vi "Dust_Source_Control_small.vi"(7 "error in":errorcluster) -> (0 "error out":errorcluster)   [LabVIEW 2013]
doc: "This VI specifies the properties of the pulse used for running the dust source. When program is stopped, the voltage is incrementally reduced to zero to avoid quick drops."
uses:
  <vilib>/Utility/miscctls.llb/LVPointTypeDef.ctl
  Global Variables/Action Items.ctl
  <vilib>/Utility/error.llb/DialogType.ctl
  <vilib>/DAQmx/read.llb/DAQmx Read (Analog 1D Wfm NChan NSamp).vi
  <vilib>/Analysis/baseanly.llb/Mean (DBL).vi
  <vilib>/DAQmx/write.llb/DAQmx Write (Analog 1D Wfm NChan NSamp).vi
  <vilib>/DAQmx/read.llb/DAQmx Read (Counter U32 1Chan 1Samp).vi
  <vilib>/DAQmx/create/channels.llb/DAQmx Create Channel (AI-Voltage-Basic).vi
  <vilib>/DAQmx/configure/timing.llb/DAQmx Timing (Sample Clock).vi
  <vilib>/DAQmx/create/channels.llb/DAQmx Create Channel (AO-Voltage-Basic).vi
  <vilib>/DAQmx/create/channels.llb/DAQmx Create Channel (CI-Count Edges).vi
  <userlib>/_OpenG.lib/comparison/comparison.llb/DBL Changed__ogtk.vi
  <vilib>/measure/mascope.llb/Amplitude and Levels 1 chan.vi
  <vilib>/DAQmx/miscellaneous.llb/DAQmx Fill In Error Info.vi
  Global Variables/throttle.vi
  <userlib>/_OpenG.lib/comparison/comparison.llb/Boolean Changed__ogtk.vi
  Global Variables/throttle from query.vi
  Sub-Polymorphic/post_run_times.vi
  Sub-Polymorphic/update_counter_entry_small.vi
  Sub-Polymorphic/post_dust_event_big.vi
  Sub-Polymorphic/post_dust_source_small.vi
  <vilib>/addons/database/_DB Variant To Data/Database Variant To Data.xnode
  <resource>/objmgr/daqmx.rc
  <vilib>/measure/NI_MAPro.lvlib
  <vilib>/Analysis/NI_AALBase.lvlib
panel:
  out "Freq. Before Throttle":dbl
  out "On/Off":bool
  out "Finished":bool=TRUE
  out "Output waveform":waveform(dbl)={"t0"=timestamp(0 s since 1904-01-01), "dt"=4e-06, "Y"=array[50000 elements]}
  out "Input waveform":waveform(dbl)={"t0"=timestamp(3437998856.0330505 s since 1904-01-01), "dt"=0.00019999999999999998, "Y"=array[1000 elements], "attributes"=variant("NI_ChannelName"=variant(string "Dev5/ai20"), "NI_UnitDescription"=variant(string "Volts"))}
  out "output cluster":T1={"Integer Timestamp"=0, "Needle Voltage"=0.0, "Frequency"=1.0, "Width (ms) : 0.1 "=0.1, "Desired Amplitude (V)"=0.0, "Settings ID"="", "ID#"=0} {"Needle Voltage" min=0.0 max=10.0 step=0.01 format="%.2g"; "Desired Amplitude (V)" min=0.0 max=10.0 step=0.01 format="%5.2f"; "Width (ms) : 0.1" min=0.05 max=5.0 step=0.01 format="%6.2f"; "Frequency" min=1.0 max=100.0 step=0.01 format="%.1f"}
  in  "Tab Control":enum32{"Controls", "Status", "Counter"}(tab)
  in  "Big Accelerator\nSetting?":bool
  out "Actual output width (ms)":dbl caption="Actual Output Width (ms)" format="%.2f"
  out "Actual output Frequency":dbl caption="Actual Output  Frequency (hz)" format="%.2f"
  in  "Width (ms) : 0.1":dbl=0.1 min=0.0 max=5.0 step=0.01 format="%6.2f"
  out "Actual Amplitude (V) 2":dbl=0.0012999050305587314 caption="Actual Amplitude (V)" format="%.2f"
  in  "Desired Amplitude (V)":dbl min=0.0 max=10.0 step=0.01 format="%5.2f"
  out "Actual output Amplitude (V)":dbl caption="Actual Output Amplitude (V)" format="%.2f"
  in  "Frequency":dbl=1.0 caption="Frequency (Hz) : 1" min=0.0 max=30.0 step=0.01 format="%.1f"
  in  "Abort Change":bool
  out "Actual Needle (kV)":dbl=-1.1093266413053247 caption="Actual Einzel (V)" format="%.2f"
  out "Actual Needle Output (V)":dbl caption="Actual Einzel (V)" format="%.2f"
  in  "Needle Voltage":dbl min=0.0 max=10.0 step=0.01 format="%.2g"
  in  "Save Settings?":bool
  out "CONTROLS":waveform(dbl)[](graph)=[{"t0"=timestamp(0 s since 1904-01-01), "dt"=4e-06, "Y"=array[50000 elements]}, {"t0"=timestamp(3437998856.0330505 s since 1904-01-01), "dt"=0.00019999999999999998, "Y"=array[1000 elements], "attributes"=variant("NI_ChannelName"=variant(string "Dev5/ai20"), "NI_UnitDescription"=variant(string "Volts"))}]
  in  "Settings ID":string
  in  "Retrieve Settings":bool
  out "Ratio of particles at\nsecond detector to first":dbl
  out "First detector since\nlast source change:":i64
  out "Average Rate of first":dbl
  out "Average Rate of second":dbl
  in  "# of Cycles ot Average":i32=10
  out "Number of Hours":dbl
  out "Chamber Pressure":dbl format="%#_3g"
  in  "Physical Channels":tag="Dev4/ao0:1" caption="Physical Output Channels"
  in  "Physical Input Channels":tag="Dev6/ai0:2"
  out "Execution Number:":i32=341
  out "Testing":bool
  in  "Counters On/Off":bool=TRUE
  in  "Reset Counters":bool
  in  "Det1":tag="Dev5/ctr0"
  in  "Det2":tag="Dev5/ctr1"
  out "Det2":u32
  out "Det1":u32
  out "error?":bool
  out "Actual Sample Clock Rate":dbl=250000.0 format="%.2f"
  in  "stop":bool
  # "CCLDAS Dust Control Small Accelerator"
  # "Hold Down to\nStop Changes"
  # "Tube Drive (Ao0, Ai4)"
  # "Needle Control (Ao4, Ai0)"
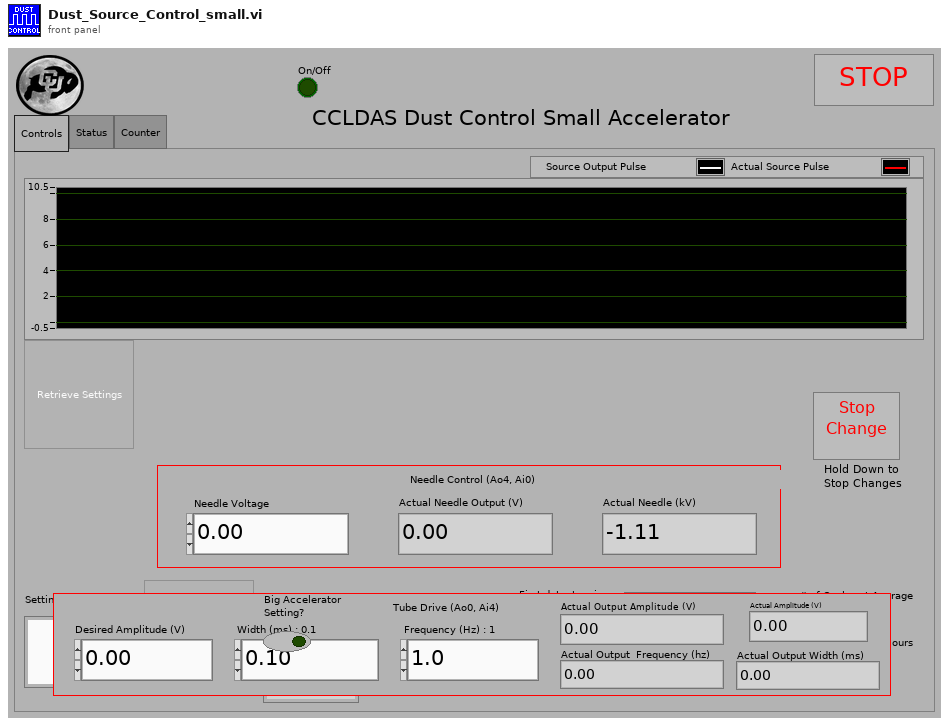
[diagram p1: front panel]
types:
  T1 = cluster{"Integer Timestamp":u64, "Needle Voltage":dbl, "Frequency":dbl, "Width (ms) : 0.1 ":dbl, "Desired Amplitude (V)":dbl, "Settings ID":string, "ID#":i32}
  T2 = typedef "Action Items.ctl" = enum16{"Initialize", "Get", "Set"}
  T3 = typedef "LVPointTypeDef.ctl" = cluster{"Horizontal":i16, "Vertical":i16}
  T4 = enum8{"Enabled", "Disabled", "Disabled and Grayed Out"}
  T5 = typedef "DialogType.ctl" = u16
  T6 = typedef "dust_source_control.ctl" = cluster{"Integer Timestamp":u64, "Einzel Voltage":dbl, "Needle Voltage":dbl, "Frequency":dbl, "Width (ms) : 0.1 ":dbl, "Desired Amplitude (V)":dbl, "X Voltage":dbl, "Y Voltage":dbl, "Settings ID":string, "ID#":i32}
  T7 = cluster{"Integer Time":i64, "Integer Time":i64, "Experiment ID":i64}
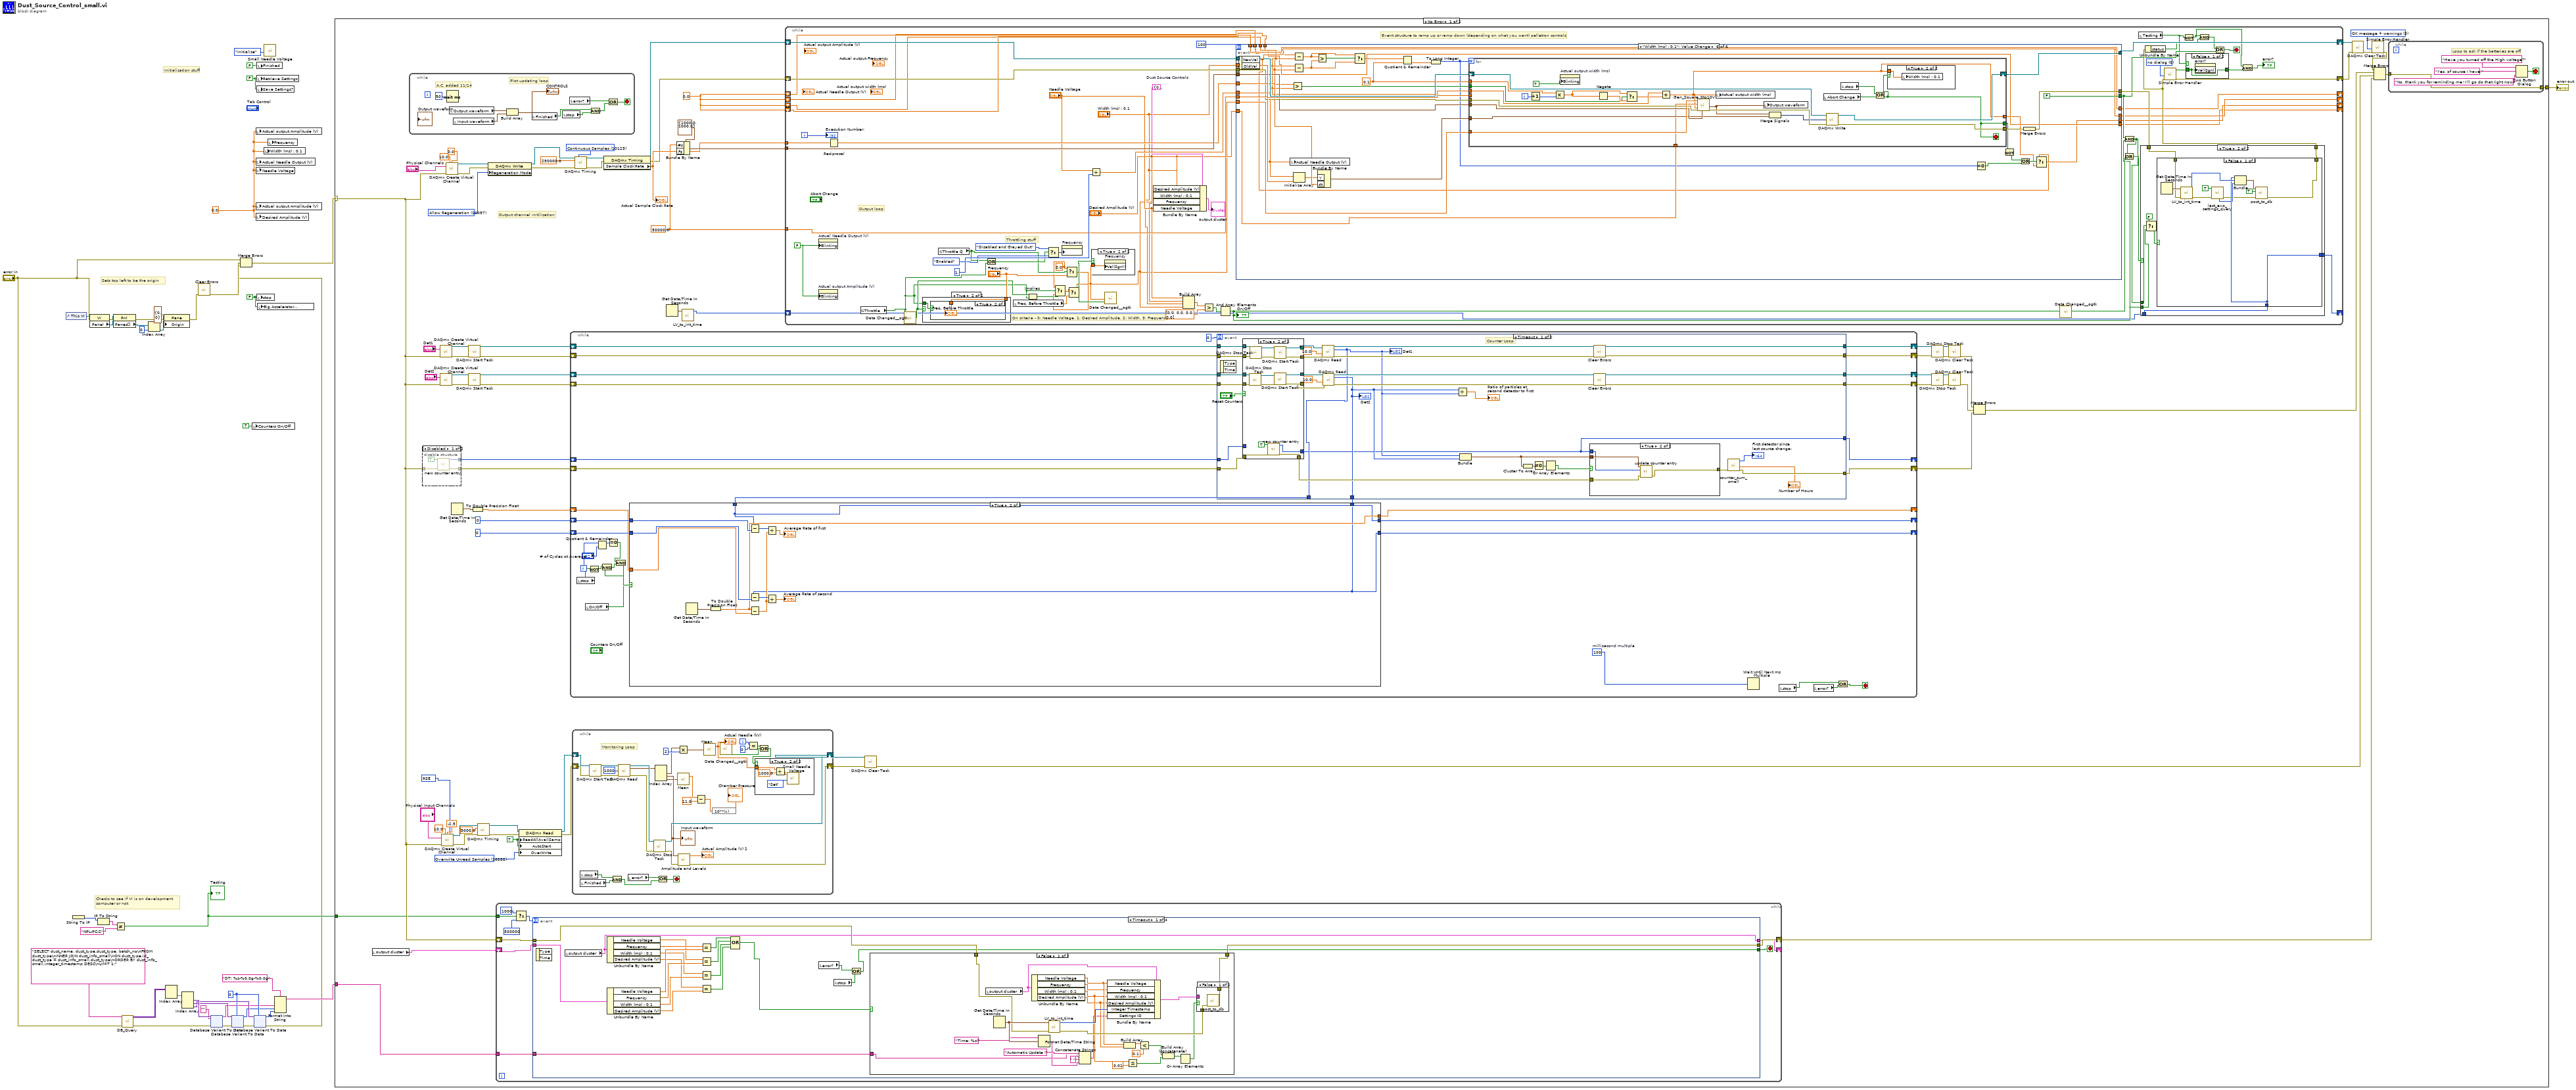
[diagram p0: block diagram]
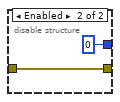
[diagram p2: hidden frame]
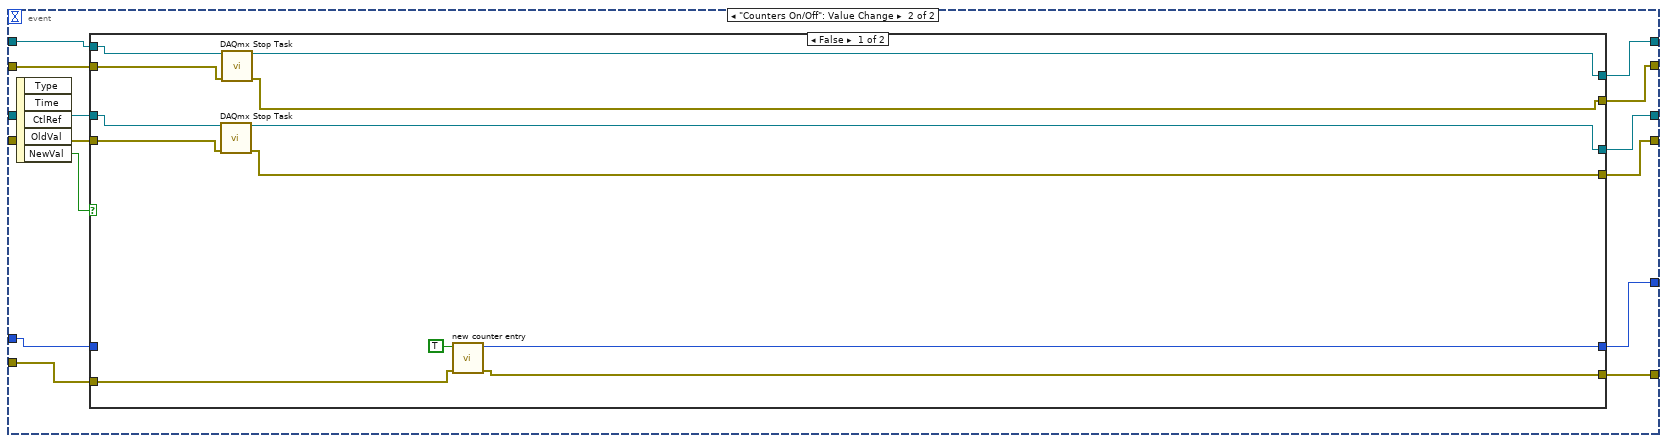
[diagram p5: hidden frame]
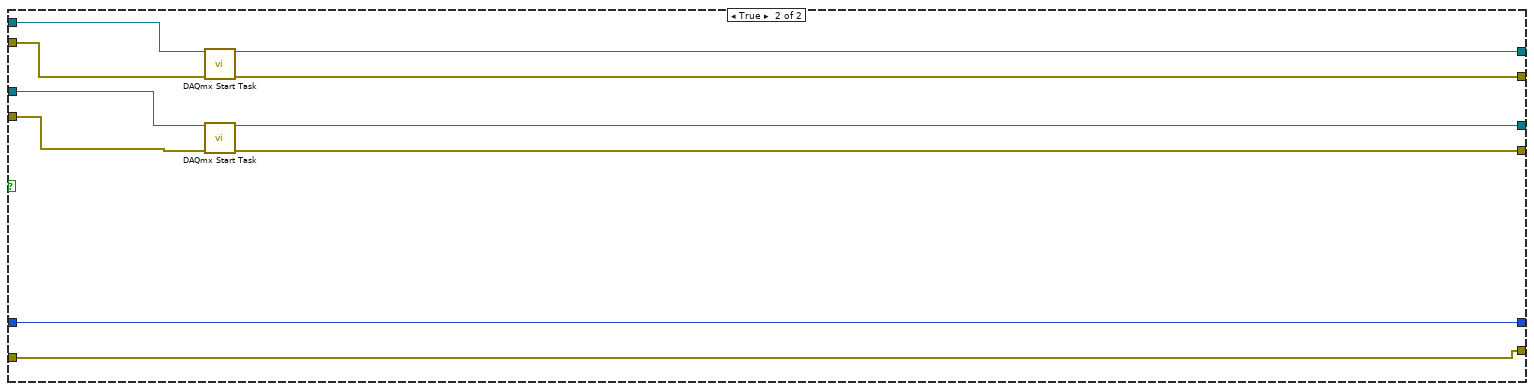
[diagram p6: hidden frame]
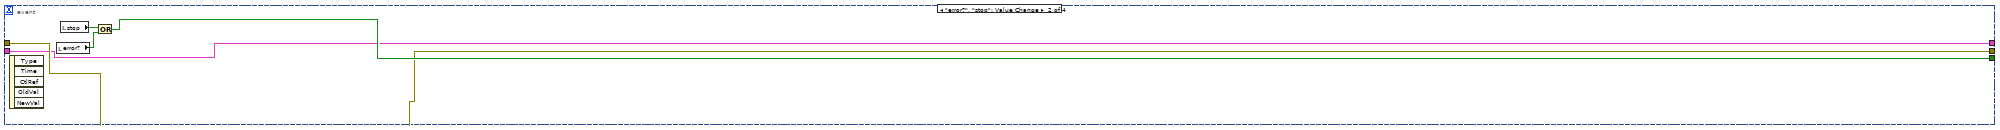
[diagram p11: hidden frame]
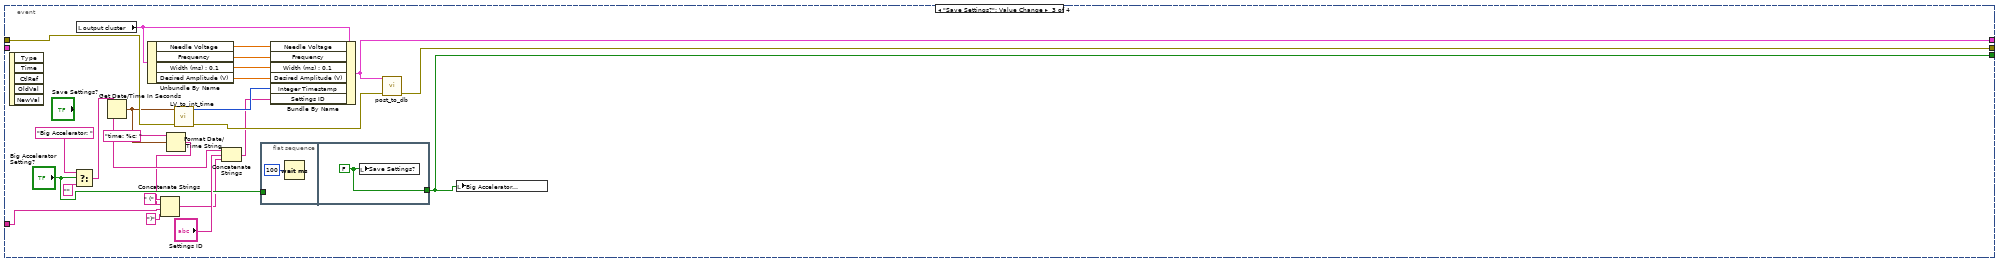
[diagram p12: hidden frame]
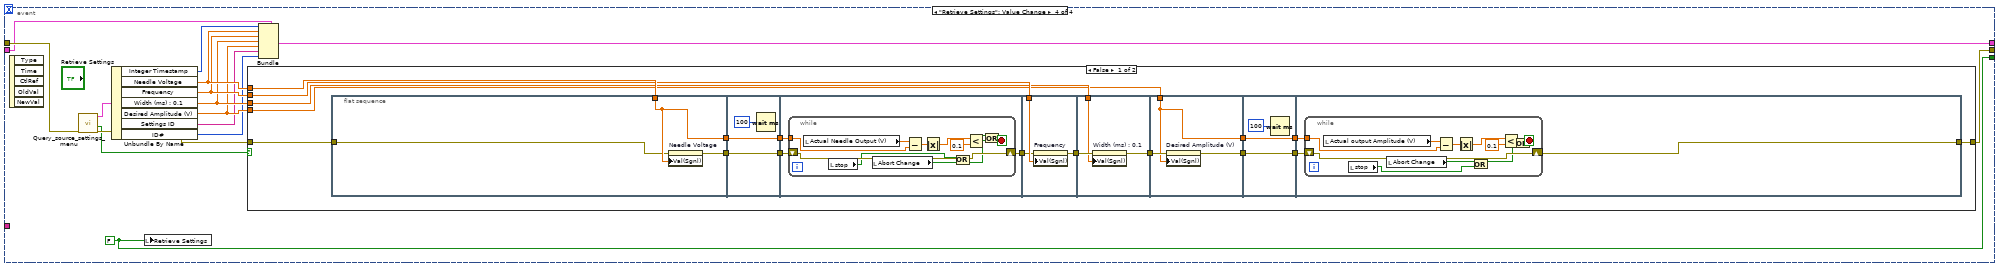
[diagram p13: hidden frame]
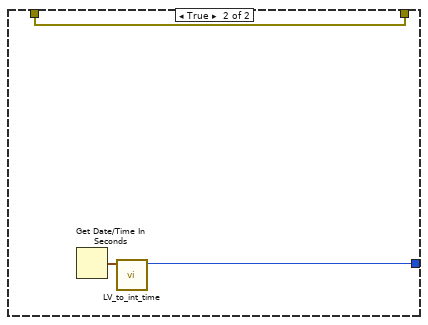
[diagram p19: hidden frame]
diagram:
  w16 = 0
  w38 = FALSE ("Retrieve Settings")
  w36 = 0.0 ("Actual Output (V)")
  w35 = FALSE ("Shutdown")
  # "Checks to see if VI is on development\ncomputer or not"
  # "Sets top left to be the origin"
  # "Initialization stuff"
  n1 = control-ref of="This VI"() -> (w34:refnum<vi>)
  n2 = String To IP() -> (0:w26:u32)  [unwired: 1 in]
  n3 = property class="VI"(reference=w34, error in="error in") -> (error out=w33:errorcluster, "Panel"=w32:refnum<vi>)  [unwired: 1 out]
  n4 = IP To String(2:w26) -> (0:w25:string)  [unwired: 1 in]
  n5 = property class="Pnl"(reference=w32, error in=w33) -> (error out=w31:errorcluster, "Panes[]"=w30:refnum<vi>[])  [unwired: 1 out]
  n6 = Not Equal?(x=w25, y="NPL-PC-2") -> (x != y?=w10:bool)
  "Testing" <- w10
  n7 = call "DB_Query.vi"("error in (no error)"="error in", "Parameterized Query"="SELECT dust_name, dust_type.dust_type, batch_no\nFROM dust_type\nINNER JOIN dust_info_small\nON dust_type.id_dust_type = dust_info_small.dust_type\nORDER BY dust_info_small.integer_timestamp DESC\nLIMIT 1;" ("SQL query")) -> ("error out"=w4:errorcluster, "Results"=w3:variant[][])  [unwired: 7 in, 1 out]
  n8 = Index Array(array=w30, index=0) -> (element=w28:refnum<vi>)
  n9 = property class="Pane"(reference=w28, error in=w31, "Origin"=T3 {"Horizontal"=0, "Vertical"=0}) -> (error out=w7:errorcluster)  [unwired: 1 out]
  n10 = Index Array(array=w3) -> (element=w23:variant[])  [unwired: 2 in]
  n11 = Index Array(array=w23) -> (element #1=w22:variant, element #2=w19:variant, element #3=w18:variant)  [unwired: 3 in]
  n12 = call <vilib>:"Clear Errors.vi"("error in (no error)"=w7) -> ("error out"=w8:errorcluster)  [unwired: 6 in]
  n13 = xnode "Database Variant To Data"("database variant"=w22, "error in (no error)"=w4, "type"="") -> ("data"=w14:string, "error out"=w21:errorcluster)
  n14 = xnode "Database Variant To Data"("database variant"=w19, "error in (no error)"=w21, "type"=w16) -> ("data"=w13:i32, "error out"=w20:errorcluster)
  n15 = local write "Counters On/Off"(TRUE ("Counters On/Off")) -> ()
  n16 = xnode "Database Variant To Data"("database variant"=w18, "error in (no error)"=w20, "type"=w16) -> ("data"=w12:i32, "error out"=w5:errorcluster)
  n17 = Merge Errors("error in", w8, w5) -> (w9:errorcluster)
  n18 = local write "Actual output Amplitude (V)"(w36) -> ()
  n19 = local write "Actual Needle Output (V)"(w36) -> ()
  n20 = local write "Needle Voltage"(w36) -> ()
  n21 = local write "Actual output Amplitude (V)"(w36) -> ()
  n22 = local write "Desired Amplitude (V)"(w36) -> ()
  n23 = local write "Finished"(FALSE ("Finished")) -> ()
  n24 = local write "Retrieve Settings"(w38) -> ()
  n25 = local write "Save Settings?"(w38) -> ()
  n26 = local write "stop"(w35) -> ()
  n27 = local write "Big Accelerator\nSetting?"(w35) -> ()
  n28 = local write "Width (ms) : 0.1"(w36) -> ()
  n29 = call "Small Needle Voltage.vi"("Action"=Action_Items."Initialize") -> ()  [unwired: 10 in, 1 out]
  n30 = local write "Frequency"(w36) -> ()
  n31 = Format Into String(format string="DT: %s-%0.0g-%0.0g", w14, w13, w12) -> (resulting string=w11:string)  [unwired: 2 in, 1 out]
  n32 = case shown="No Error" w9 {
    selector: w9 -> [w53 w924]
    tunnel: [w95 w924] -> w40
    tunnel: w11 -> [w43 _]
    tunnel: w10 -> [w42 _]
    frame No Error {
      w41 = 10083 items=["default"=-1, "RSE"=10083, "NRSE"=10078, "Differential"=10106, "Pseudodifferential"=12529] ("input terminal configuration")
      w50 = 0.0 ("Width (ms) : 3.5")
      w63 = 10252 items=["Overwrite Unread Samples"=10252, "Do Not Overwrite Unread Samples"=10159] ("OverWrite")
      w64 = TRUE ("ReadAllAvailSamp")
      w46 = 50000.0 ("Size (Samples)")
      w108 = 10097 items=["Allow Regeneration"=10097, "Do Not Allow Regeneration"=10158] ("RegenMode")
      w113 = T5 3 items=["no dialog", "OK message", "continue or stop message", "OK message + warnings", "continue/stop + warnings"] ("type of dialog (OK msg:1)")
      w117 = 10123 items=["Finite Samples"=10178, "Continuous Samples"=10123] ("sample mode")
      # "Output channel initilization"
      n33 = local read "output cluster"() -> (w45:T1)
      n34 = while {
        stop <- w279 stop-if-true
        # "Plot updating loop"
        # "A.C. added 11/14"
        n35 = Wait (ms)(milliseconds to wait=u32 50) -> ()  [unwired: 1 out]
        n36 = local read "Output waveform"() -> (w276:waveform(dbl))
        n37 = local read "Input waveform"() -> (w277:waveform(dbl))
        n38 = Build Array(w276, w277) -> (→"CONTROLS":waveform(dbl)[])
        n39 = local read "Finished"() -> (w274:bool)
        n40 = local read "stop"() -> (w275:bool)
        n41 = local read "error?"() -> (w278:bool)
        n42 = And(x=w274, y=w275) -> (x .and. y?=w273:bool)
        n43 = Or(x=w278, y=w273) -> (x .or. y?=w279:bool)
      }
      n44 = disable-structure shown="Disabled" {
        disable-tunnel: [w121 w123] -> w72
        disable-tunnel: [w120 i64 0 ("Integer Time")] -> w71
        disable-tunnel: w53 -> [w119 w123]
        frame Disabled {
          n45 = call "new counter entry.vi"("error in"=w119, "Small?"=TRUE) -> ("error out"=w121:errorcluster, "Integer Time"=w120:i64)  [unwired: 8 in]
        }
        frame Enabled {
        }
      }
      n46 = call-poly <vilib>:"DAQmx Create Virtual Channel.vi"("counter"="Det1", "error in"=w53) -> ("task out"=w80:refnum<k21>, "error out"=w77:errorcluster)  [unwired: 12 in]
      n47 = call-poly <vilib>:"DAQmx Create Virtual Channel.vi"("counter"="Det2", "error in"=w53) -> ("task out"=w79:refnum<k21>, "error out"=w78:errorcluster)  [unwired: 12 in]
      n48 = call-poly <vilib>:"DAQmx Create Virtual Channel.vi"("maximum value"=10.0 ("Maximum Value"), "minimum value"=-2.5 ("Minimum Value"), "input terminal configuration"=w41, "physical channels"="Physical Input Channels", "error in"=w53) -> ("task out"=w57:refnum<k21>, "error out"=w56:errorcluster)  [unwired: 9 in]
      n49 = call-poly <vilib>:"DAQmx Create Virtual Channel.vi"("maximum value"=10.0 ("Maximum Value"), "minimum value"=0.0 ("Minimum Value"), "physical channels"="Physical Channels", "error in"=w53) -> ("task out"=w107:refnum<k21>, "error out"=w106:errorcluster)  [unwired: 10 in]
      n50 = Get Date/Time In Seconds() -> (seconds since 1Jan1904=w70:timestamp)
      n51 = call <vilib>:"DAQmx Start Task.vi"("task/channels in"=w80, "error in"=w77) -> ("task out"=w92:refnum<k21>, "error out"=w89:errorcluster)  [unwired: 12 in]
      n52 = call <vilib>:"DAQmx Start Task.vi"("task/channels in"=w79, "error in"=w78) -> ("task out"=w91:refnum<k21>, "error out"=w90:errorcluster)  [unwired: 12 in]
      n53 = To Double Precision Float(number=w70) -> (double precision float=w69:dbl)
      n54 = call-poly <vilib>:"DAQmx Timing.vi"("task/channels in"=w57, "rate"=5000.0, "error in"=w56) -> ("task out"=w62:refnum<k21>, "error out"=w61:errorcluster)  [unwired: 11 in]
      n55 = property class="DAQmx Write"(reference=w107, error in=w106, "Regeneration Mode"=w108) -> (reference out=w105:refnum<k21>, error out=w104:errorcluster)
      n56 = while {
        shift-right: [w325] -> w74
        shift-left: w53 -> [w324]
        shift-right: [w317] -> _
        shift-left: w45 -> [w326]
        tunnel: w42 -> [w320]
        tunnel: w43 -> [w318]
        stop <- w323 stop-if-true
        n57 = Select(t=1000, s=w320, f=300000) -> (s? t:f=w322:i32)
        n58 = event shown="[0] Timeout" {
          selector: _ -> [_ _ _ _]
          dyn-events: _ -> [_ _ _ _]
          timeout: w322 -> [_ _ _ _]
          tunnel: [w327 w376 w381 w407] -> w317
          tunnel: w326 -> [w347 w376 _ w415]
          tunnel: [w332 w377 w404 w421] -> w325
          tunnel: w324 -> [w333 w377 w401 w419]
          tunnel: [w330 w378 w390 w420] -> w323
          tunnel: w318 -> [w334 _ w387 _]
          event Timeout {
            n59 = event-data() -> ()  [unwired: 1 in, 2 out]
            n60 = local read "output cluster"() -> (w327:T1)
            n61 = Unbundle By Name(w327) -> ("Needle Voltage"=w346:dbl, "Frequency"=w344:dbl, "Width (ms) : 0.1"=w342:dbl, "Desired Amplitude (V)"=w340:dbl)
            n62 = Unbundle By Name(w347) -> ("Needle Voltage"=w345:dbl, "Frequency"=w343:dbl, "Width (ms) : 0.1"=w335:dbl, "Desired Amplitude (V)"=w341:dbl)
            n63 = Equal?(x=w346, y=w345) -> (x = y?=w339:bool)
            n64 = Equal?(x=w344, y=w343) -> (x = y?=w338:bool)
            n65 = Equal?(x=w342, y=w335) -> (x = y?=w337:bool)
            n66 = Equal?(x=w340, y=w341) -> (x = y?=w336:bool)
            n67 = Compound Arithmetic op=OR(w339, w338, w337, w336) -> (w331:bool)
            n68 = local read "error?"() -> (w329:bool)
            n69 = local read "stop"() -> (w328:bool)
            n70 = Or(x=w329, y=w328) -> (x .or. y?=w330:bool)
            n71 = case shown="False" w331 {
              tunnel: w334 -> [w348 _]
              tunnel: w333 -> [w353 w375]
              tunnel: [w352 w375] -> w332
              frame False {
                n72 = local read "output cluster"() -> (w357:T1)
                n73 = Get Date/Time In Seconds() -> (seconds since 1Jan1904=w369:timestamp)
                n74 = Unbundle By Name(w357) -> ("Needle Voltage"=w367:dbl, "Frequency"=w363:dbl, "Width (ms) : 0.1"=w362:dbl, "Desired Amplitude (V)"=w366:dbl)
                n75 = Format Date/Time String(time format string (%c)="Time: %c)" ("Settings ID"), seconds (now)=w369) -> (date/time string=w349:string)  [unwired: 1 in]
                n76 = call "LV_to_int_time.vi"("error in (no error)"=w353, "Time Stamp"=w369) -> ("error out"=w370:errorcluster, "Integer Time"=w371:i64)  [unwired: 7 in]
                n77 = Concatenate Strings("Automatic Update (" ("string"), w348, " " ("string"), w349) -> (w355:string)
                n78 = Bundle By Name(cluster=w357, "Needle Voltage"=w367, "Frequency"=w363, "Width (ms) : 0.1"=w362, "Desired Amplitude (V)"=w366, "Integer Timestamp"=w371, "Settings ID"=w355) -> (w358:T1)
                n79 = Build Array(w367, w366) -> (w365:dbl[])
                n80 = Less Or Equal?(x=w362, y=0.01) -> (x <= y?=w356:bool)
                n81 = Less?(x=w365, y=0.1) -> (x < y?=w360:bool[])
                n82 = Build Array (concatenate)(w360, w356) -> (w359:bool[])
                n83 = Or Array Elements(Boolean array=w359) -> (logical OR=w354:bool)
                n84 = case shown="False" w354 {
                  tunnel: w358 -> [_ _]
                  tunnel: [w373 w374] -> w352
                  tunnel: w370 -> [w372 w374]
                  frame False {
                    n85 = call-poly "post_to_db.vi"("error in (no error)"=w372) -> ("error out"=w373:errorcluster)  [unwired: 8 in, 2 out]
                  }
                  frame True {
                  }
                }
              }
              frame True {
              }
            }
          }
          event "error?", "stop": Value Change {
            n86 = event-data() -> ()  [unwired: 1 in, 5 out]
            n87 = local read "error?"() -> (w379:bool)
            n88 = local read "stop"() -> (w380:bool)
            n89 = Or(x=w380, y=w379) -> (x .or. y?=w378:bool)
          }
          event "Save Settings?": Value Change {
            n90 = event-data() -> ()  [unwired: 1 in, 5 out]
            n91 = Select(t="Big Accelerator: ", s="Big Accelerator\nSetting?", f="") -> (s? t:f=w392:string)
            n92 = local read "output cluster"() -> (w382:T1)
            n93 = Get Date/Time In Seconds() -> (seconds since 1Jan1904=w399:timestamp)
            n94 = Unbundle By Name(w382) -> ("Needle Voltage"=w398:dbl, "Frequency"=w397:dbl, "Width (ms) : 0.1"=w396:dbl, "Desired Amplitude (V)"=w395:dbl)
            n95 = Format Date/Time String(time format string (%c)="time: %c; " ("Settings ID"), seconds (now)=w399) -> (date/time string=w385:string)  [unwired: 1 in]
            n96 = Concatenate Strings(" (" ("string"), w385, w387, ")" ("string")) -> (w384:string)
            n97 = call "LV_to_int_time.vi"("error in (no error)"=w401, "Time Stamp"=w399) -> ("error out"=w402:errorcluster, "Integer Time"=w403:i64)  [unwired: 7 in]
            n98 = Concatenate Strings(w392, "Settings ID", w384) -> (w383:string)
            n99 = flat-sequence {
              tunnel: "Big Accelerator\nSetting?" -> [_]
              tunnel: [w406] -> w390
              frame #0 {
                n100 = Wait (ms)(milliseconds to wait=u32 100) -> ()  [unwired: 1 out]
              }
              frame #1 {
                w406 = FALSE
                n101 = local write "Save Settings?"(w406) -> ()
              }
            }
            n102 = Bundle By Name(cluster=w382, "Needle Voltage"=w398, "Frequency"=w397, "Width (ms) : 0.1"=w396, "Desired Amplitude (V)"=w395, "Integer Timestamp"=w403, "Settings ID"=w383) -> (w381:T1)
            n103 = call-poly "post_to_db.vi"("error in (no error)"=w402, "Dust control settings"=w381) -> ("error out"=w404:errorcluster)  [unwired: 9 in]
            n104 = local write "Big Accelerator\nSetting?"(w390) -> ()
          }
          event "Retrieve Settings": Value Change {
            w420 = FALSE
            n105 = event-data() -> ()  [unwired: 1 in, 5 out]
            n106 = call "Query_source_settings_menu.vi"("error in (no error)"=w419) -> ("error out"=w417:errorcluster, "Cancelled?"=w416:bool, "Output cluster"=w418:T6)  [unwired: 8 in]
            n107 = Unbundle By Name(w418) -> ("Integer Timestamp"=w410:u64, "Needle Voltage"=w414:dbl, "Frequency"=w413:dbl, "Width (ms) : 0.1"=w412:dbl, "Desired Amplitude (V)"=w411:dbl, "Settings ID"=w409:string, "ID#"=w408:i32)
            n108 = local write "Retrieve Settings"(w420) -> ()
            n109 = case shown="False" w416 {
              tunnel: w417 -> [w438 w485]
              tunnel: w414 -> [w437 _]
              tunnel: w413 -> [w436 _]
              tunnel: w412 -> [w434 _]
              tunnel: w411 -> [w425 _]
              tunnel: [w422 w485] -> w421
              frame False {
                n110 = flat-sequence {
                  tunnel: w437 -> [w440]
                  tunnel: [w441] -> w433
                  tunnel: [w440] -> w429
                  tunnel: w438 -> [w439]
                  tunnel: w433 -> [w444]
                  tunnel: [w444] -> w432
                  tunnel: [w442] -> w430
                  tunnel: w429 -> [w442]
                  tunnel: w432 -> [w446]
                  tunnel: w430 -> [w447]
                  tunnel: [w445] -> w428
                  tunnel: w436 -> [w461]
                  tunnel: [w460] -> w435
                  tunnel: w428 -> [w459]
                  tunnel: w435 -> [w464]
                  tunnel: w434 -> [w462]
                  tunnel: [w463] -> w427
                  tunnel: w427 -> [w467]
                  tunnel: [w465] -> w426
                  tunnel: w425 -> [w466]
                  tunnel: [w466] -> w424
                  tunnel: w426 -> [w470]
                  tunnel: [w470] -> w431
                  tunnel: w424 -> [w468]
                  tunnel: [w468] -> w423
                  tunnel: [w473] -> w422
                  tunnel: w431 -> [w472]
                  tunnel: w423 -> [w471]
                  frame #0 {
                    n111 = property on="Needle Voltage" class="DigNum (strict)"(error in=w439, "Val(Sgnl)"=w440) -> (error out=w441:errorcluster)  [unwired: 1 in, 1 out]
                  }
                  frame #1 {
                    n112 = Wait (ms)(milliseconds to wait=u32 100) -> ()  [unwired: 1 out]
                  }
                  frame #2 {
                    n113 = while {
                      tunnel: w447 -> [w453]
                      shift-right: [w458] -> w445
                      shift-left: w446 -> [w458]
                      stop <- w451 stop-if-true
                      n114 = local read "Actual Needle Output (V)"() -> (w454:dbl)
                      n115 = local read "stop"() -> (w448:bool)
                      n116 = local read "Abort Change"() -> (w450:bool)
                      n117 = Subtract(x=w454, y=w453) -> (x-y=w457:dbl)
                      n118 = Absolute Value(x=w457) -> (abs(x)=w456:dbl)
                      n119 = Or(x=w448, y=w450) -> (x .or. y?=w449:bool)
                      n120 = Less?(x=w456, y=0.1) -> (x < y?=w452:bool)
                      n121 = Or(x=w449, y=w452) -> (x .or. y?=w451:bool)
                    }
                  }
                  frame #3 {
                    n122 = property on="Frequency" class="DigNum (strict)"(error in=w459, "Val(Sgnl)"=w461) -> (error out=w460:errorcluster)  [unwired: 1 in, 1 out]
                  }
                  frame #4 {
                    n123 = property on="Width (ms) : 0.1" class="DigNum (strict)"(error in=w464, "Val(Sgnl)"=w462) -> (error out=w463:errorcluster)  [unwired: 1 in, 1 out]
                  }
                  frame #5 {
                    n124 = property on="Desired Amplitude (V)" class="DigNum (strict)"(error in=w467, "Val(Sgnl)"=w466) -> (error out=w465:errorcluster)  [unwired: 1 in, 1 out]
                  }
                  frame #6 {
                    n125 = Wait (ms)(milliseconds to wait=u32 100) -> ()  [unwired: 1 out]
                  }
                  frame #7 {
                    n126 = while {
                      tunnel: w471 -> [w484]
                      shift-right: [w482] -> w473
                      shift-left: w472 -> [w482]
                      stop <- w477 stop-if-true
                      n127 = local read "Actual output Amplitude (V)"() -> (w483:dbl)
                      n128 = local read "stop"() -> (w474:bool)
                      n129 = local read "Abort Change"() -> (w475:bool)
                      n130 = Subtract(x=w483, y=w484) -> (x-y=w480:dbl)
                      n131 = Absolute Value(x=w480) -> (abs(x)=w479:dbl)
                      n132 = Or(x=w475, y=w474) -> (x .or. y?=w476:bool)
                      n133 = Less?(x=w479, y=0.1) -> (x < y?=w481:bool)
                      n134 = Or(x=w481, y=w476) -> (x .or. y?=w477:bool)
                    }
                  }
                }
              }
              frame True {
              }
            }
            n135 = Bundle(cluster=w415, "Integer Timestamp"=w410, "Needle Voltage"=w414, "Frequency"=w413, "Width (ms) : 0.1"=w412, "Desired Amplitude (V)"=w411, "Settings ID"=w409, "ID#"=w408) -> (w407:T1)
          }
        }
      }
      n136 = property class="DAQmx Read"(reference=w62, error in=w61, "ReadAllAvailSamp"=w64, "AutoStart"=w64, "OverWrite"=w63) -> (reference out=w54:refnum<k21>, error out=w52:errorcluster)
      n137 = while {
        shift-right: [w143] -> _
        shift-left: w71 -> [w145]
        shift-right: [w138] -> _
        shift-left: w69 -> [w134]
        shift-right: [w137] -> _
        shift-left: u32 0 ("data") -> [w141]
        shift-right: [w136] -> _
        shift-left: u32 0 ("data") -> [w140]
        shift-right: [w157] -> w88
        shift-left: w92 -> [w149]
        shift-right: [w151] -> w87
        shift-left: w89 -> [w148]
        shift-right: [w156] -> w86
        shift-left: w91 -> [w147]
        shift-right: [w155] -> w85
        shift-left: w90 -> [w146]
        shift-right: [w150] -> w47
        shift-left: w72 -> [w144]
        i -> [w126]
        stop <- w152 stop-if-true
        w154 = u32 100  # millisecond multiple
        n138 = local read "stop"() -> (w133:bool)
        n139 = local read "On/Off"() -> (w125:bool)
        n140 = Not(x=w133) -> (.not. x?=w132:bool)
        n141 = Quotient & Remainder(x=w126, y="# of Cycles ot Average") -> (x-y*floor(x/y)=w135:i32)  [unwired: 1 out]
        n142 = And(x=w132, y=w125) -> (x .and. y?=w129:bool)
        n143 = Equal To 0?(x=w135) -> (x = 0?=w130:bool)
        n144 = And(x=w130, y=w129) -> (x .and. y?=w131:bool)
        n145 = event shown="[0] Timeout" {
          selector: _ -> [_ _]
          dyn-events: _ -> [_ _]
          timeout: 0 -> [_ _]
          tunnel: [w189 w226] -> w157
          tunnel: [w186 w224] -> w156
          tunnel: [w185 w223] -> w155
          tunnel: [w181 w225] -> w151
          tunnel: [w180 w217] -> w150
          tunnel: w149 -> [w178 w221]
          tunnel: w148 -> [w177 w228]
          tunnel: w147 -> [w176 w222]
          tunnel: w146 -> [w175 w227]
          tunnel: w145 -> [w169 w220]
          tunnel: w144 -> [w168 w218]
          tunnel: [w159 w219] -> w143
          tunnel: [w165 _] -> w139
          tunnel: [w160 _] -> w124
          event Timeout {
            # "Counter Loop"
            n146 = event-data() -> ()  [unwired: 1 in, 2 out]
            n147 = case shown="True" "Reset Counters" {
              tunnel: w178 -> [w200 w216]
              tunnel: [w200 w214] -> w174
              tunnel: w177 -> [w199 w213]
              tunnel: [w199 w211] -> w173
              tunnel: w176 -> [w198 w210]
              tunnel: [w198 w208] -> w172
              tunnel: w175 -> [w197 w207]
              tunnel: [w197 w205] -> w171
              tunnel: w168 -> [w196 w203]
              tunnel: [w195 w204] -> w159
              tunnel: [w196 w202] -> w167
              tunnel: w169 -> [w195 _]
              frame False {
              }
              frame True {
                n148 = call <vilib>:"DAQmx Stop Task.vi"("task/channels in"=w210, "error in"=w207) -> ("task out"=w209:refnum<k21>, "error out"=w206:errorcluster)  [unwired: 12 in]
                n149 = call <vilib>:"DAQmx Stop Task.vi"("task/channels in"=w216, "error in"=w213) -> ("task out"=w215:refnum<k21>, "error out"=w212:errorcluster)  [unwired: 12 in]
                n150 = call "new counter entry.vi"("error in"=w203, "Small?"=TRUE) -> ("error out"=w202:errorcluster, "Integer Time"=w204:i64)  [unwired: 8 in]
                n151 = call <vilib>:"DAQmx Start Task.vi"("task/channels in"=w209, "error in"=w206) -> ("task out"=w208:refnum<k21>, "error out"=w205:errorcluster)  [unwired: 12 in]
                n152 = call <vilib>:"DAQmx Start Task.vi"("task/channels in"=w215, "error in"=w212) -> ("task out"=w214:refnum<k21>, "error out"=w211:errorcluster)  [unwired: 12 in]
              }
            }
            n153 = call-poly <vilib>:"DAQmx Read.vi"("task/channels in"=w174, "timeout"=10.0, "error in"=w173) -> ("task out"=w189:refnum<k21>, "data"=w165:u32, "error out"=w184:errorcluster)  [unwired: 10 in]
            "Det1" <- w165
            n154 = call-poly <vilib>:"DAQmx Read.vi"("task/channels in"=w172, "timeout"=10.0, "error in"=w171) -> ("task out"=w186:refnum<k21>, "data"=w160:u32, "error out"=w183:errorcluster)  [unwired: 10 in]
            "Det2" <- w160
            n155 = Divide(x=w160, y=w165) -> (x/y=→"Ratio of particles at\nsecond detector to first":dbl)
            n156 = Bundle("data"=w165, "data"=w160) -> (w158:cluster{"data":u32, "data":u32})  [unwired: 1 in]
            n157 = Cluster To Array(cluster=w158) -> (array=w164:u32[])
            n158 = Not Equal To 0?(x=w164) -> (x != 0?=w163:bool[])
            n159 = Or Array Elements(Boolean array=w163) -> (logical OR=w162:bool)
            n160 = case shown="True" w162 {
              tunnel: [w190 w191] -> w179
              tunnel: w167 -> [w190 w192]
              tunnel: w159 -> [_ w193]
              tunnel: w158 -> [_ w194]
              frame False {
              }
              frame True {
                n161 = call-poly "update counter entry.vi"("error in"=w192, "Integer Time"=w193, "input cluster"=w194) -> ("error out"=w191:errorcluster)  [unwired: 8 in]
              }
            }
            n162 = call <vilib>:"Clear Errors.vi"("error in (no error)"=w184) -> ("error out"=w181:errorcluster)  [unwired: 6 in]
            n163 = call <vilib>:"Clear Errors.vi"("error in (no error)"=w183) -> ("error out"=w185:errorcluster)  [unwired: 6 in]
            n164 = call "counter_sum_small.vi"("error in"=w179) -> ("error IO"=w180:errorcluster, "Number of Hours"=→"Number of Hours":dbl, "First Detector Sum"=→"First detector since\nlast source change:":i64)  [unwired: 7 in, 1 out]
          }
          event "Counters On/Off": Value Change {
            n165 = event-data() -> ("NewVal"=w229:bool)  [unwired: 1 in, 4 out]
            n166 = case shown="False" w229 {
              tunnel: w228 -> [w240 w247]
              tunnel: w227 -> [w238 w246]
              tunnel: [w234 w251] -> w226
              tunnel: [w235 w250] -> w225
              tunnel: [w236 w249] -> w224
              tunnel: [w237 w248] -> w223
              tunnel: w222 -> [w239 w245]
              tunnel: w221 -> [w241 w244]
              tunnel: w220 -> [_ w243]
              tunnel: [w233 w243] -> w219
              tunnel: w218 -> [w232 w242]
              tunnel: [w231 w242] -> w217
              frame False {
                n167 = call <vilib>:"DAQmx Stop Task.vi"("task/channels in"=w239, "error in"=w238) -> ("task out"=w236:refnum<k21>, "error out"=w237:errorcluster)  [unwired: 12 in]
                n168 = call <vilib>:"DAQmx Stop Task.vi"("task/channels in"=w241, "error in"=w240) -> ("task out"=w234:refnum<k21>, "error out"=w235:errorcluster)  [unwired: 12 in]
                n169 = call "new counter entry.vi"("error in"=w232, "Small?"=TRUE) -> ("error out"=w231:errorcluster, "Integer Time"=w233:i64)  [unwired: 8 in]
              }
              frame True {
                n170 = call <vilib>:"DAQmx Start Task.vi"("task/channels in"=w244, "error in"=w247) -> ("task out"=w251:refnum<k21>, "error out"=w250:errorcluster)  [unwired: 12 in]
                n171 = call <vilib>:"DAQmx Start Task.vi"("task/channels in"=w245, "error in"=w246) -> ("task out"=w249:refnum<k21>, "error out"=w248:errorcluster)  [unwired: 12 in]
              }
            }
          }
        }
        n172 = case shown="True" w131 {
          tunnel: w134 -> [w254 w265]
          tunnel: w141 -> [w253 w264]
          tunnel: w140 -> [w252 w263]
          tunnel: w139 -> [_ w258]
          tunnel: [w254 w259] -> w138
          tunnel: [w253 w258] -> w137
          tunnel: [w252 w255] -> w136
          tunnel: w124 -> [_ w255]
          frame False {
          }
          frame True {
            n173 = Get Date/Time In Seconds() -> (seconds since 1Jan1904=w266:timestamp)
            n174 = To Double Precision Float(number=w266) -> (double precision float=w259:dbl)
            n175 = Subtract(x=w258, y=w264) -> (x-y=w262:u32)
            n176 = Subtract(x=w255, y=w263) -> (x-y=w261:u32)
            n177 = Subtract(x=w259, y=w265) -> (x-y=w260:dbl)
            n178 = Divide(x=w262, y=w260) -> (x/y=→"Average Rate of first":dbl)
            n179 = Divide(x=w261, y=w260) -> (x/y=→"Average Rate of second":dbl)
          }
        }
        n180 = Wait Until Next ms Multiple(millisecond multiple=w154) -> ()  [unwired: 1 out]
        n181 = local read "stop"() -> (w127:bool)
        n182 = local read "error?"() -> (w153:bool)
        n183 = Or(x=w127, y=w153) -> (x .or. y?=w152:bool)
      }
      n184 = while {
        shift-right: [w293] -> w51
        shift-left: w54 -> [w295]
        shift-right: [w296] -> w66
        shift-left: w52 -> [w294]
        i -> [w283]
        stop <- w297 stop-if-true
        # "Monitoring Loop"
        n185 = local read "stop"() -> (w311:bool)
        n186 = local read "Finished"() -> (w312:bool)
        n187 = call <vilib>:"DAQmx Start Task.vi"("task/channels in"=w295, "error in"=w294) -> ("task out"=w302:refnum<k21>, "error out"=w303:errorcluster)  [unwired: 12 in]
        n188 = And(x=w311, y=w312) -> (x .and. y?=w310:bool)
        n189 = call-poly <vilib>:"DAQmx Read.vi"("task/channels in"=w302, "number of samples per channel"=1000, "error in"=w303) -> ("task out"=w304:refnum<k21>, "data"=w298:waveform(dbl)[], "error out"=w305:errorcluster)  [unwired: 10 in]
        n190 = local read "error?"() -> (w299:bool)
        n191 = call <vilib>:"DAQmx Stop Task.vi"("task/channels in"=w304, "error in"=w305) -> ("task out"=w293:refnum<k21>, "error out"=w309:errorcluster)  [unwired: 12 in]
        n192 = Index Array(array=w298) -> (element #1=w300:waveform(dbl), element #2=w292:waveform(dbl), element #3=w291:waveform(dbl))  [unwired: 3 in]
        "Input waveform" <- w292
        n193 = Or(x=w299, y=w310) -> (x .or. y?=w297:bool)
        n194 = Multiply(x=w300, y=2) -> (x*y=w306:waveform(dbl))
        n195 = call-poly <vilib>:"Mean.vi"("X"=w291) -> ("mean"=w290:dbl)  [unwired: 1 out]
        n196 = call-poly <vilib>:"Amplitude and Levels.vi"("error in (no error)"=w309, "signal in"=w292) -> ("error out"=w296:errorcluster, "amplitude"=→"Actual Amplitude (V) 2":dbl)  [unwired: 6 in, 2 out]
        n197 = Subtract(x=w290, y=11.0) -> (x-y=w288:dbl)
        n198 = call-poly <vilib>:"Mean.vi"("X"=w306) -> ("mean"=w286:dbl)  [unwired: 1 out]
        "Actual Needle (kV)" <- w286
        n199 = expression code="10**(x)"(w288) -> (→"Chamber Pressure":dbl)
        n200 = call-poly <userlib>:"Data Changed__ogtk.vi"("DBL"=w286) -> ("Changed"=w284:bool)
        n201 = Equal?(x=w283, y=0) -> (x = y?=w281:bool)
        n202 = Or(x=w281, y=w284) -> (x .or. y?=w285:bool)
        n203 = case shown="True" w285 {
          tunnel: w286 -> [_ w314]
          frame False {
          }
          frame True {
            n204 = Divide(x=w314, y=1000.0) -> (x/y=w315:dbl)
            n205 = call "Small Needle Voltage.vi"("Action"=Action_Items."Set", "Input Pelletron Voltage"=w315) -> ()  [unwired: 9 in, 1 out]
          }
        }
      }
      n206 = call-poly <vilib>:"DAQmx Timing.vi"("task/channels in"=w105, "sample mode"=w117, "rate"=250000.0 ("Sample Clock Rate"), "error in"=w104) -> ("task out"=w111:refnum<k21>, "error out"=w97:errorcluster)  [unwired: 10 in]
      n207 = property class="DAQmx Timing"(reference=w111, error in=w97) -> (reference out=w99:refnum<k21>, error out=w44:errorcluster, "Sample Clock:Rate"=w103:dbl)
      "Actual Sample Clock Rate" <- w103
      n208 = Get Date/Time In Seconds() -> (seconds since 1Jan1904=w49:timestamp)
      n209 = Bundle By Name(cluster=cluster{"Fs":dbl, "#s":dbl} {"Fs"=1000.0, "#s"=1000.0} ("sampling info"), "#s"=w46, "Fs"=w103) -> (w109:cluster{"Fs":dbl, "#s":dbl})
      n210 = call "LV_to_int_time.vi"("Time Stamp"=w49) -> ("Integer Time"=w48:i64)  [unwired: 8 in, 1 out]
      n211 = while {
        tunnel: w109 -> [w545]
        tunnel: w103 -> [w543]
        tunnel: w46 -> [w532]
        shift-right: [w542] -> w102
        shift-left: w99 -> [w540]
        shift-right: [w539] -> w98
        shift-left: w44 -> [w547]
        shift-right: [w501] -> _
        shift-left: w50 -> [w505]
        shift-right: [w500] -> _
        shift-left: w50 -> [w504]
        shift-right: [w499] -> _
        shift-left: w50 -> [w503]
        shift-right: [w498] -> _
        shift-left: w50 -> [w502]
        shift-right: [w494] -> _
        shift-left: w48 -> [w495]
        i -> [w546]
        stop <- w488 stop-if-true
        w526 = 0.0 ("t")
        w534 = T1 {"Integer Timestamp"=0, "Needle Voltage"=1.0, "Frequency"=0.0, "Width (ms) : 0.1 "=0.0, "Desired Amplitude (V)"=0.0, "Settings ID"="", "ID#"=0}  # Dust Source Controls
        w538 = T5 0 items=["no dialog", "OK message", "continue or stop message", "OK message + warnings", "continue/stop + warnings"] ("type of dialog (OK msg:1)")
        w537 = FALSE ("Blinking")
        # "On criteria - 0: Needle Voltage, 1: Desired Amplitude, 2: Width, 3: Frequency"
        # "Event structure to ramp up or ramp down (depending on what you want) pelletron controls"
        # "Throttling stuff"
        # "Output loop"
        n212 = property on="Actual Needle Output (V)" class="DigNum (strict)"("Blinking"=w537) -> ()  [unwired: 2 in, 2 out]
        n213 = property on="Actual output Amplitude (V)" class="DigNum (strict)"("Blinking"=w537) -> ()  [unwired: 2 in, 2 out]
        n214 = Reciprocal(x=w543) -> (1/x=w544:dbl)
        n215 = global read "throttle.vi" "Throttle"() -> (w506:bool)
        n216 = call-poly <userlib>:"Data Changed__ogtk.vi"("Boolean"=w506) -> ("Changed"=w508:bool)
        n217 = case shown="True" w508 {
          tunnel: w506 -> [_ w551]
          tunnel: "Frequency" -> [_ w550]
          frame False {
          }
          frame True {
            n218 = case shown="True" w551 {
              tunnel: w550 -> [_ w552]
              frame False {
              }
              frame True {
                "Freq. Before Throttle" <- w552
              }
            }
          }
        }
        n219 = global read "throttle from query.vi" "Throttle Q"() -> (w527:bool)
        n220 = Or(x=w527, y=w506) -> (x .or. y?=w528:bool)
        n221 = local read "Freq. Before Throttle"() -> (w509:dbl)
        n222 = Implies(1:w506, 2:w508) -> (0:w507:bool)
        n223 = Select(t=T4."Disabled and Grayed Out" ("Disabled"), s=w528, f=T4."Enabled" ("Disabled")) -> (s? t:f=w529:T4)
        n224 = property on="Frequency" class="DigNum (strict)"("DisabledEnum"=w529) -> ()  [unwired: 2 in, 2 out]
        n225 = Select(t=w526, s=w527, f="Frequency") -> (s? t:f=w524:dbl)
        n226 = Select(t=w526, s=w506, f=w524) -> (s? t:f=w520:dbl)
        n227 = Select(t=w520, s=w507, f=w509) -> (s? t:f=w510:dbl)
        n228 = Divide(x="Needle Voltage", y=1) -> (x/y=w536:dbl)
        n229 = call-poly <userlib>:"Data Changed__ogtk.vi"("DBL"=w510) -> ("Changed"=w525:bool)
        n230 = case shown="True" w525 {
          tunnel: w510 -> [_ w577]
          frame False {
          }
          frame True {
            n231 = property on="Frequency" class="DigNum (strict)"("Val(Sgnl)"=w577) -> ()  [unwired: 2 in, 2 out]
          }
        }
        n232 = Bundle By Name(cluster=w534, "Desired Amplitude (V)"="Desired Amplitude (V)", "Width (ms) : 0.1"="Width (ms) : 0.1", "Frequency"=w510, "Needle Voltage"="Needle Voltage") -> (→"output cluster":T1)
        n233 = Build Array("Needle Voltage", "Desired Amplitude (V)", "Width (ms) : 0.1", w510) -> (w519:dbl[])
        n234 = Greater?(x=w519, y=dbl[] [0.0, 0.0, 0.0, 0.0]) -> (0:w517:bool[])
        n235 = And Array Elements(Boolean array=w517) -> (logical AND=w496:bool)
        "On/Off" <- w496
        n236 = event shown="[5] \"Width (ms) : 0.1\": Value Change" {
          selector: _ -> [_ _ _ _ _ _]
          dyn-events: _ -> [_ _ _ _ _ _]
          timeout: 100 -> [_ _ _ _ _ _]
          tunnel: w545 -> [w587 w629 w693 w777 w836 w895]
          tunnel: w547 -> [w602 w624 w692 w762 w821 w880]
          tunnel: w510 -> [w582 w638 w694 w779 w838 w897]
          tunnel: "Width (ms) : 0.1" -> [w583 w639 w695 w780 w839 w898]
          tunnel: [w601 w623 w680 w760 w819 w878] -> w516
          tunnel: w540 -> [w600 w637 w687 w778 w837 w896]
          tunnel: "Desired Amplitude (V)" -> [w585 w621 w676 _ w818 w877]
          tunnel: w532 -> [w591 w634 w690 w774 w833 w892]
          tunnel: w544 -> [w590 w633 w691 w773 w832 w891]
          tunnel: [w594 w636 w688 w776 w835 w894] -> w542
          tunnel: [FALSE ("y") FALSE ("y") TRUE ("y") FALSE ("y") FALSE ("y") FALSE ("y")] -> w513
          tunnel: w536 -> [w589 _ w682 w770 w829 w888]
          tunnel: w505 -> [w581 w620 _ w758 w816 w875]
          tunnel: w504 -> [w580 w619 _ w759 w815 w874]
          tunnel: w503 -> [w579 w618 _ w757 w814 w876]
          tunnel: w502 -> [w578 w617 _ w756 w817 w873]
          tunnel: [w581 w611 w675 w758 w816 w875] -> w501
          tunnel: [w580 w619 w675 w750 w815 w874] -> w500
          tunnel: [w579 w618 w675 w757 w814 w867] -> w499
          tunnel: [w578 w617 w675 w756 w806 w873] -> w498
          event Timeout {
            w584 = FALSE ("Blinking")
            n237 = event-data() -> ()  [unwired: 1 in, 2 out]
            n238 = local write "Actual Needle Output (V)"(w589) -> ()
            n239 = local write "Actual output Amplitude (V)"(w585) -> ()
            n240 = call "Gen_Square_0to10V.vi"("sampling info"=w587, "error in (no error)"=w602, "Width (ms)"=w583, "amplitude"=w585, "frequency"=w582) -> ("error out"=w597:errorcluster, "signal out"=w586:waveform(dbl))  [unwired: 5 in]
            n241 = Initialize Array(w589, w591) -> (w592:dbl[])
            n242 = local write "Actual output width (ms)"(w583) -> ()
            n243 = local write "Actual output Frequency"(w582) -> ()
            n244 = local write "Output waveform"(w586) -> ()
            n245 = Bundle By Name("Y"=w592, "dt"=w590) -> (w588:waveform(dbl))  [unwired: 1 in]
            n246 = Merge Signals(w586, w588) -> (w595:dynamicdata)
            n247 = call-poly <vilib>:"DAQmx Write.vi"("task/channels in"=w600, "data"=w595, "error in"=w597) -> ("task out"=w599:refnum<k21>, "error out"=w596:errorcluster)  [unwired: 10 in, 1 out]
            n248 = First Call?() -> (First Call?: T/F=w598:bool)
            n249 = case shown="True" w598 {
              tunnel: [w603 w608] -> w601
              tunnel: [w604 w607] -> w594
              tunnel: w599 -> [w604 w606]
              tunnel: w596 -> [w603 w605]
              frame False {
              }
              frame True {
                n250 = call <vilib>:"DAQmx Start Task.vi"("task/channels in"=w606, "error in"=w605) -> ("task out"=w607:refnum<k21>, "error out"=w608:errorcluster)  [unwired: 12 in]
              }
            }
            n251 = property on="Actual output Amplitude (V)" class="DigNum (strict)"("Blinking"=w584) -> ()  [unwired: 2 in, 2 out]
            n252 = property on="Actual Needle Output (V)" class="DigNum (strict)"("Blinking"=w584) -> ()  [unwired: 2 in, 2 out]
            n253 = property on="Actual output width (ms)" class="DigNum (strict)"("Blinking"=w584) -> ()  [unwired: 2 in, 2 out]
            n254 = property on="Actual output Frequency" class="DigNum (strict)"("Blinking"=w584) -> ()  [unwired: 2 in, 2 out]
          }
          event "Needle Voltage": Value Change {
            (unwired) "needle" ("name (unnamed)")
            w630 = 0.05 ("y")
            n255 = event-data() -> ("NewVal"=w610:dbl)  [unwired: 1 in, 4 out]
            n256 = Greater?(x=w610, y=w620) -> (0:w632:bool)
            n257 = Subtract(x=w610, y=w620) -> (x-y=w626:dbl)
            n258 = Subtract(x=w620, y=w610) -> (x-y=w627:dbl)
            n259 = Greater?(x=w626, y=w627) -> (0:w628:bool)
            n260 = Select(t=w626, s=w628, f=w627) -> (s? t:f=w625:dbl)
            n261 = Divide(x=w625, y=w630) -> (x/y=w631:dbl)
            n262 = To Long Integer(number=w631) -> (32bit integer=w609:i32)
            n263 = for {
              N: w609 -> [_]
              tunnel: w630 -> [w670]
              tunnel: w620 -> [w669]
              tunnel: w633 -> [w667]
              tunnel: w634 -> [w666]
              tunnel: [w649] -> w622
              tunnel: w639 -> [w647]
              tunnel: w621 -> [w648]
              tunnel: w638 -> [w662]
              tunnel: w624 -> [w661]
              shift-right: [w665] -> w636
              shift-left: w637 -> [w660]
              tunnel: w632 -> [w654]
              tunnel: w629 -> [w653]
              tunnel: [w643] -> w612
              tunnel: [w641] -> w613
              i -> [w671]
              stop <- w641 stop-if-true
              n264 = local write "Actual output Amplitude (V)"(w648) -> ()
              n265 = call "Gen_Square_0to10V.vi"("sampling info"=w653, "error in (no error)"=w661, "Width (ms)"=w647, "amplitude"=w648, "frequency"=w662) -> ("error out"=w663:errorcluster, "signal out"=w650:waveform(dbl))  [unwired: 5 in]
              n266 = Increment(x=w671) -> (x+1=w672:i32)
              n267 = property on="Actual Needle Output (V)" class="DigNum (strict)"("Blinking"=TRUE) -> ()  [unwired: 2 in, 2 out]
              n268 = local write "Output waveform"(w650) -> ()
              n269 = Multiply(x=w670, y=w672) -> (x*y=w656:dbl)
              n270 = Negate(x=w656) -> (-x=w657:dbl)
              n271 = Select(t=w656, s=w654, f=w657) -> (s? t:f=w655:dbl)
              n272 = Add(x=w669, y=w655) -> (x+y=w652:dbl)
              n273 = Divide(x=w652, y=1.0) -> (x/y=w645:dbl)
              n274 = Less Than 0?(x=w645) -> (x < 0?=w646:bool)
              n275 = Select(t=0.0, s=w646, f=w645) -> (s? t:f=w643:dbl)
              n276 = local write "Actual Needle Output (V)"(w643) -> ()
              n277 = Initialize Array(w643, w666) -> (w668:dbl[])
              n278 = Bundle By Name("Y"=w668, "dt"=w667) -> (w658:waveform(dbl))  [unwired: 1 in]
              n279 = Merge Signals(w650, w658) -> (w664:dynamicdata)
              n280 = local read "Abort Change"() -> (w642:bool)
              n281 = local read "stop"() -> (w640:bool)
              n282 = call-poly <vilib>:"DAQmx Write.vi"("task/channels in"=w660, "data"=w664, "error in"=w663) -> ("task out"=w665:refnum<k21>, "error out"=w649:errorcluster)  [unwired: 10 in, 1 out]
              n283 = Or(x=w642, y=w640) -> (x .or. y?=w641:bool)
              n284 = case shown="True" w641 {
                tunnel: w643 -> [_ w673]
                frame False {
                }
                frame True {
                  n285 = local write "Needle Voltage"(w673) -> ()
                }
              }
            }
            n286 = Equal To 0?(x=w609) -> (x = 0?=w615:bool)
            n287 = Not(x=w613) -> (.not. x?=w616:bool)
            n288 = Merge Errors(w622) -> (w623:errorcluster)
            n289 = Or(x=w616, y=w615) -> (x .or. y?=w614:bool)
            n290 = Select(t=w610, s=w614, f=w612) -> (s? t:f=w611:dbl)
          }
          event "stop": Value Change {
            w675 = 0.0 ("Width (ms) : 3.5")
            w679 = TRUE ("Blinking")
            n291 = event-data() -> ()  [unwired: 1 in, 1 out]
            n292 = property on="Actual Needle Output (V)" class="DigNum (strict)"("Blinking"=w679) -> ()  [unwired: 2 in, 2 out]
            n293 = property on="Actual output Amplitude (V)" class="DigNum (strict)"("Blinking"=w679) -> ()  [unwired: 2 in, 2 out]
            n294 = Multiply(x=w682, y=20.0 ("x")) -> (x*y=w684:dbl)
            n295 = Multiply(x=20.0, y=w676) -> (x*y=w674:dbl)
            n296 = Greater?(x=w684, y=w674) -> (0:w683:bool)
            n297 = Select(t=w684, s=w683, f=w674) -> (s? t:f=w677:dbl)
            n298 = Increment(x=w677) -> (x+1=w678:dbl)
            n299 = for {
              N: w678 -> [w703]
              tunnel: w695 -> [w716]
              tunnel: w694 -> [w715]
              tunnel: w693 -> [w709]
              tunnel: w676 -> [w717]
              tunnel: w690 -> [w707]
              tunnel: w691 -> [w706]
              tunnel: [w706] -> _ mode=indexing
              shift-right: [w711] -> w681
              shift-left: w692 -> [w710]
              tunnel: w682 -> [w699]
              tunnel: w687 -> [w713]
              tunnel: [w714] -> w688
              i -> [w705]
              n300 = Subtract(x=w703, y=1) -> (x-y=w702:i32)
              n301 = Wait (ms)(milliseconds to wait=u32 250) -> ()  [unwired: 1 out]
              n302 = Equal?(x=w702, y=w705) -> (x = y?=w704:bool)
              n303 = case shown="True" w704 {
                tunnel: w717 -> [w740 _]
                tunnel: w716 -> [w739 _]
                tunnel: w715 -> [w738 _]
                tunnel: [w737 w746] -> w712
                tunnel: w710 -> [w736 w746]
                tunnel: w709 -> [w732 _]
                tunnel: [w731 w747] -> w708
                tunnel: w703 -> [w728 _]
                tunnel: w707 -> [w724 w742]
                tunnel: w706 -> [w726 w744]
                tunnel: w705 -> [w718 _]
                tunnel: w699 -> [w727 _]
                tunnel: [w720 w745] -> w698
                frame False {
                  n304 = Divide(x=w727, y=w728) -> (x/y=w730:dbl)
                  n305 = Divide(x=w740, y=w728) -> (x/y=w735:dbl)
                  n306 = Multiply(x=w730, y=w718) -> (x*y=w729:dbl)
                  n307 = Multiply(x=w735, y=w718) -> (x*y=w734:dbl)
                  n308 = Subtract(x=w727, y=w729) -> (x-y=w721:dbl)
                  n309 = Subtract(x=w740, y=w734) -> (x-y=w733:dbl)
                  n310 = local write "Actual output Amplitude (V)"(w733) -> ()
                  n311 = call "Gen_Square_0to10V.vi"("sampling info"=w732, "error in (no error)"=w736, "Width (ms)"=w739, "amplitude"=w733, "frequency"=w738) -> ("error out"=w737:errorcluster, "signal out"=w720:waveform(dbl))  [unwired: 5 in]
                  n312 = Divide(x=w721, y=1.0) -> (x/y=w722:dbl)
                  n313 = local write "Actual Needle Output (V)"(w722) -> ()
                  n314 = Initialize Array(w722, w724) -> (w725:dbl[])
                  n315 = Bundle By Name("Y"=w725, "dt"=w726) -> (w719:waveform(dbl))  [unwired: 1 in]
                  n316 = Merge Signals(w720, w719) -> (w731:dynamicdata)
                }
                frame True {
                  w743 = 0.0 ("element")
                  n317 = local write "Actual Needle Output (V)"(w743) -> ()
                  n318 = local write "Needle Voltage"(w743) -> ()
                  n319 = local write "Desired Amplitude (V)"(w743) -> ()
                  n320 = local write "Actual output Amplitude (V)"(w743) -> ()
                  n321 = Initialize Array(w743, w742) -> (w741:dbl[])
                  n322 = Bundle By Name("Y"=w741, "dt"=w744) -> (w745:waveform(dbl))  [unwired: 1 in]
                  n323 = Merge Signals(w745, w745) -> (w747:dynamicdata)
                }
              }
              n324 = local write "Output waveform"(w698) -> ()
              n325 = call-poly <vilib>:"DAQmx Write.vi"("task/channels in"=w713, "data"=w708, "error in"=w712) -> ("task out"=w714:refnum<k21>, "error out"=w711:errorcluster)  [unwired: 10 in, 1 out]
            }
            n326 = flat-sequence {
              tunnel: w681 -> [w697]
              tunnel: [w697] -> w680
              frame #0 {
                w696 = TRUE ("Finished")
                n327 = local write "stop"(w696) -> ()
                "Finished" <- w696
              }
            }
          }
          event "Desired Amplitude (V)": Value Change {
            w767 = 0.05 ("y")
            n328 = event-data() -> ("NewVal"=w749:dbl)  [unwired: 1 in, 1 out]
            n329 = local write "Actual Needle Output (V)"(w770) -> ()
            n330 = Greater?(x=w749, y=w759) -> (0:w769:bool)
            n331 = Subtract(x=w749, y=w759) -> (x-y=w765:dbl)
            n332 = Subtract(x=w759, y=w749) -> (x-y=w763:dbl)
            n333 = Initialize Array(w770, w774) -> (w772:dbl[])
            n334 = Greater?(x=w765, y=w763) -> (0:w766:bool)
            n335 = Bundle By Name("Y"=w772, "dt"=w773) -> (w771:waveform(dbl))  [unwired: 1 in]
            n336 = Select(t=w765, s=w766, f=w763) -> (s? t:f=w764:dbl)
            n337 = Quotient & Remainder(x=w764, y=w767) -> (floor(x/y)=w768:dbl)  [unwired: 1 out]
            n338 = To Long Integer(number=w768) -> (32bit integer=w748:i32)
            n339 = for {
              N: w748 -> [_]
              tunnel: w780 -> [w803]
              tunnel: w779 -> [w802]
              tunnel: w759 -> [w800]
              tunnel: w762 -> [w799]
              tunnel: [w797] -> w761
              tunnel: w777 -> [w795]
              tunnel: w767 -> [w792]
              tunnel: w771 -> [w790]
              shift-right: [w796] -> w776
              shift-left: w778 -> [w798]
              tunnel: w769 -> [w786]
              tunnel: [w784] -> w751
              tunnel: [w782] -> w752
              i -> [w801]
              stop <- w782 stop-if-true
              n340 = Increment(x=w801) -> (x+1=w794:i32)
              n341 = property on="Actual output Amplitude (V)" class="DigNum (strict)"("Blinking"=TRUE) -> ()  [unwired: 2 in, 2 out]
              n342 = Multiply(x=w792, y=w794) -> (x*y=w787:dbl)
              n343 = Negate(x=w787) -> (-x=w789:dbl)
              n344 = Select(t=w787, s=w786, f=w789) -> (s? t:f=w788:dbl)
              n345 = Add(x=w800, y=w788) -> (x+y=w784:dbl)
              n346 = local write "Actual output Amplitude (V)"(w784) -> ()
              n347 = call "Gen_Square_0to10V.vi"("sampling info"=w795, "error in (no error)"=w799, "Width (ms)"=w803, "amplitude"=w784, "frequency"=w802) -> ("error out"=w804:errorcluster, "signal out"=w785:waveform(dbl))  [unwired: 5 in]
              n348 = local write "Output waveform"(w785) -> ()
              n349 = Merge Signals(w785, w790) -> (w791:dynamicdata)
              n350 = call-poly <vilib>:"DAQmx Write.vi"("task/channels in"=w798, "data"=w791, "error in"=w804) -> ("task out"=w796:refnum<k21>, "error out"=w797:errorcluster)  [unwired: 10 in, 1 out]
              n351 = local read "Abort Change"() -> (w783:bool)
              n352 = local read "stop"() -> (w781:bool)
              n353 = Or(x=w783, y=w781) -> (x .or. y?=w782:bool)
              n354 = case shown="True" w782 {
                tunnel: w784 -> [_ w805]
                frame False {
                }
                frame True {
                  n355 = local write "Desired Amplitude (V)"(w805) -> ()
                }
              }
            }
            n356 = Equal To 0?(x=w748) -> (x = 0?=w754:bool)
            n357 = Not(x=w752) -> (.not. x?=w755:bool)
            n358 = Merge Errors(w761) -> (w760:errorcluster)
            n359 = Or(x=w755, y=w754) -> (x .or. y?=w753:bool)
            n360 = Select(t=w749, s=w753, f=w751) -> (s? t:f=w750:dbl)
          }
          event "Frequency": Value Change {
            w826 = 0.5 ("y")
            n361 = event-data() -> ("NewVal"=w808:dbl)  [unwired: 1 in, 1 out]
            n362 = local write "Actual Needle Output (V)"(w829) -> ()
            n363 = Greater?(x=w808, y=w817) -> (0:w828:bool)
            n364 = Subtract(x=w808, y=w817) -> (x-y=w824:dbl)
            n365 = Subtract(x=w817, y=w808) -> (x-y=w822:dbl)
            n366 = Initialize Array(w829, w833) -> (w831:dbl[])
            n367 = Greater?(x=w824, y=w822) -> (0:w825:bool)
            n368 = Bundle By Name("Y"=w831, "dt"=w832) -> (w830:waveform(dbl))  [unwired: 1 in]
            n369 = Select(t=w824, s=w825, f=w822) -> (s? t:f=w823:dbl)
            n370 = Quotient & Remainder(x=w823, y=w826) -> (floor(x/y)=w827:dbl)  [unwired: 1 out]
            n371 = To Long Integer(number=w827) -> (32bit integer=w807:i32)
            n372 = for {
              N: w807 -> [_]
              tunnel: w839 -> [w862]
              tunnel: w838 -> [_]
              tunnel: w817 -> [w860]
              tunnel: w821 -> [w859]
              tunnel: [w857] -> w820
              tunnel: w836 -> [w855]
              tunnel: w826 -> [w853]
              tunnel: w830 -> [w851]
              shift-right: [w856] -> w835
              shift-left: w837 -> [w858]
              tunnel: w828 -> [w847]
              tunnel: w818 -> [w844]
              tunnel: [w843] -> w809
              tunnel: [w841] -> w810
              i -> [w861]
              stop <- w841 stop-if-true
              n373 = Increment(x=w861) -> (x+1=w854:i32)
              n374 = Multiply(x=w853, y=w854) -> (x*y=w848:dbl)
              n375 = property on="Actual output Frequency" class="DigNum (strict)"("Blinking"=TRUE) -> ()  [unwired: 2 in, 2 out]
              n376 = Negate(x=w848) -> (-x=w850:dbl)
              n377 = Select(t=w848, s=w847, f=w850) -> (s? t:f=w849:dbl)
              n378 = Add(x=w860, y=w849) -> (x+y=w843:dbl)
              n379 = call "Gen_Square_0to10V.vi"("sampling info"=w855, "error in (no error)"=w859, "Width (ms)"=w862, "amplitude"=w844, "frequency"=w843) -> ("error out"=w863:errorcluster, "signal out"=w846:waveform(dbl))  [unwired: 5 in]
              n380 = local write "Actual output Frequency"(w843) -> ()
              n381 = local write "Output waveform"(w846) -> ()
              n382 = Merge Signals(w846, w851) -> (w852:dynamicdata)
              n383 = local read "Abort Change"() -> (w842:bool)
              n384 = call-poly <vilib>:"DAQmx Write.vi"("task/channels in"=w858, "data"=w852, "error in"=w863) -> ("task out"=w856:refnum<k21>, "error out"=w857:errorcluster)  [unwired: 10 in, 1 out]
              n385 = local read "stop"() -> (w840:bool)
              n386 = Or(x=w842, y=w840) -> (x .or. y?=w841:bool)
              n387 = case shown="True" w841 {
                tunnel: w843 -> [_ w864]
                frame False {
                }
                frame True {
                  n388 = local write "Frequency"(w864) -> ()
                }
              }
            }
            n389 = Equal To 0?(x=w807) -> (x = 0?=w812:bool)
            n390 = Not(x=w810) -> (.not. x?=w813:bool)
            n391 = Merge Errors(w820) -> (w819:errorcluster)
            n392 = Or(x=w813, y=w812) -> (x .or. y?=w811:bool)
            n393 = Select(t=w808, s=w811, f=w809) -> (s? t:f=w806:dbl)
          }
          event "Width (ms) : 0.1": Value Change {
            w885 = 0.1 ("y")
            n394 = event-data() -> ("NewVal"=w865:dbl)  [unwired: 1 in, 1 out]
            n395 = local write "Actual Needle Output (V)"(w888) -> ()
            n396 = Greater?(x=w865, y=w876) -> (0:w887:bool)
            n397 = Subtract(x=w865, y=w876) -> (x-y=w883:dbl)
            n398 = Subtract(x=w876, y=w865) -> (x-y=w881:dbl)
            n399 = Initialize Array(w888, w892) -> (w890:dbl[])
            n400 = Greater?(x=w883, y=w881) -> (0:w884:bool)
            n401 = Bundle By Name("Y"=w890, "dt"=w891) -> (w889:waveform(dbl))  [unwired: 1 in]
            n402 = Select(t=w883, s=w884, f=w881) -> (s? t:f=w882:dbl)
            n403 = Quotient & Remainder(x=w882, y=w885) -> (floor(x/y)=w886:dbl)  [unwired: 1 out]
            n404 = To Long Integer(number=w886) -> (32bit integer=w869:i32)
            n405 = for {
              N: w869 -> [_]
              tunnel: w898 -> [_]
              tunnel: w897 -> [w921]
              tunnel: w876 -> [w919]
              tunnel: w880 -> [w918]
              tunnel: [w916] -> w879
              tunnel: w895 -> [w914]
              tunnel: w885 -> [w912]
              tunnel: w889 -> [w910]
              shift-right: [w915] -> w894
              shift-left: w896 -> [w917]
              tunnel: w887 -> [w906]
              tunnel: w877 -> [w904]
              tunnel: [w902] -> w866
              tunnel: [w900] -> w872
              i -> [w920]
              stop <- w900 stop-if-true
              n406 = Increment(x=w920) -> (x+1=w913:i32)
              n407 = Multiply(x=w912, y=w913) -> (x*y=w907:dbl)
              n408 = property on="Actual output width (ms)" class="DigNum (strict)"("Blinking"=TRUE) -> ()  [unwired: 2 in, 2 out]
              n409 = Negate(x=w907) -> (-x=w909:dbl)
              n410 = Select(t=w907, s=w906, f=w909) -> (s? t:f=w908:dbl)
              n411 = Add(x=w919, y=w908) -> (x+y=w902:dbl)
              n412 = call "Gen_Square_0to10V.vi"("sampling info"=w914, "error in (no error)"=w918, "Width (ms)"=w902, "amplitude"=w904, "frequency"=w921) -> ("error out"=w922:errorcluster, "signal out"=w905:waveform(dbl))  [unwired: 5 in]
              n413 = local write "Actual output width (ms)"(w902) -> ()
              n414 = local write "Output waveform"(w905) -> ()
              n415 = Merge Signals(w905, w910) -> (w911:dynamicdata)
              n416 = local read "Abort Change"() -> (w901:bool)
              n417 = call-poly <vilib>:"DAQmx Write.vi"("task/channels in"=w917, "data"=w911, "error in"=w922) -> ("task out"=w915:refnum<k21>, "error out"=w916:errorcluster)  [unwired: 10 in, 1 out]
              n418 = local read "stop"() -> (w899:bool)
              n419 = Or(x=w899, y=w901) -> (x .or. y?=w900:bool)
              n420 = case shown="True" w900 {
                tunnel: w902 -> [_ w923]
                frame False {
                }
                frame True {
                  n421 = local write "Width (ms) : 0.1"(w923) -> ()
                }
              }
            }
            n422 = Equal To 0?(x=w869) -> (x = 0?=w870:bool)
            n423 = Not(x=w872) -> (.not. x?=w871:bool)
            n424 = Or(x=w871, y=w870) -> (x .or. y?=w868:bool)
            n425 = Merge Errors(w879) -> (w878:errorcluster)
            n426 = Select(t=w865, s=w868, f=w866) -> (s? t:f=w867:dbl)
          }
        }
        n427 = call-poly <userlib>:"Data Changed__ogtk.vi"("Boolean"=w496) -> ("Changed"=w497:bool)
        n428 = And(x=w513, y=w496) -> (x .and. y?=w512:bool)
        n429 = Or(x=w512, y=w497) -> (x .or. y?=w514:bool)
        n430 = local read "Testing"() -> (w492:bool)
        n431 = case shown="True" w514 {
          tunnel: w496 -> [_ w557]
          tunnel: w516 -> [w554 w562]
          tunnel: [w554 w561] -> w515
          tunnel: w512 -> [_ w556]
          tunnel: w495 -> [w553 w560]
          tunnel: [w553 w559] -> w494
          frame False {
          }
          frame True {
            n432 = Select(t=FALSE, s=w556, f=w557) -> (s? t:f=w558:bool)
            n433 = case shown="False" w558 {
              tunnel: w562 -> [w572 w576]
              tunnel: [w563 w576] -> w561
              tunnel: w560 -> [w570 _]
              tunnel: [w570 w574] -> w559
              frame False {
                n434 = Get Date/Time In Seconds() -> (seconds since 1Jan1904=w573:timestamp)
                n435 = call "LV_to_int_time.vi"("error in (no error)"=w572, "Time Stamp"=w573) -> ("error out"=w564:errorcluster, "Integer Time"=w571:i64)  [unwired: 7 in]
                n436 = call "last_exp_settings_query.vi"("error in (no error)"=w564, "Small?"=TRUE) -> ("error out"=w565:errorcluster, "Experiment ID"=w566:i64)  [unwired: 4 in, 4 out]
                n437 = Bundle("Integer Time"=w570, "Integer Time"=w571, "Experiment ID"=w566) -> (w569:T7)  [unwired: 1 in]
                n438 = call-poly "post_to_db.vi"("error in (no error)"=w565, "Small?"=TRUE, "run_times"=w569) -> ("error out"=w563:errorcluster)  [unwired: 8 in]
              }
              frame True {
                n439 = Get Date/Time In Seconds() -> (seconds since 1Jan1904=w575:timestamp)
                n440 = call "LV_to_int_time.vi"("Time Stamp"=w575) -> ("Integer Time"=w574:i64)  [unwired: 8 in, 1 out]
              }
            }
          }
        }
        n441 = Unbundle By Name(w515) -> ("status"=w491:bool)
        n442 = call <vilib>:"Simple Error Handler.vi"("type of dialog (OK msg:1)"=w538, "error in (no error)"=w515) -> ("error?"=w493:bool, "error out"=w539:errorcluster)  [unwired: 3 in, 3 out]
        n443 = Not(x=w492) -> (.not. x?=w486:bool)
        n444 = case shown="False" w492 {
          tunnel: w493 -> [w548 w549]
          tunnel: [w548 w549] -> w489
          frame False {
            n445 = property on="error?" class="Bool (strict)"("Val(Sgnl)"=w548) -> ()  [unwired: 2 in, 2 out]
          }
          frame True {
          }
        }
        n446 = And(x=w486, y=w491) -> (x .and. y?=w490:bool)
        n447 = Or(x=w490, y=w513) -> (x .or. y?=w488:bool)
        n448 = And(x=w486, y=w489) -> (x .and. y?=→"error?":bool)
        "Execution Number:" <- w546
      }
      n449 = call <vilib>:"DAQmx Clear Task.vi"("task in"=w51, "error in"=w66) -> ("error out"=w65:errorcluster)  [unwired: 13 in]
      n450 = call <vilib>:"DAQmx Stop Task.vi"("task/channels in"=w88, "error in"=w87) -> ("task out"=w84:refnum<k21>, "error out"=w83:errorcluster)  [unwired: 12 in]
      n451 = call <vilib>:"DAQmx Stop Task.vi"("task/channels in"=w86, "error in"=w85) -> ("task out"=w82:refnum<k21>, "error out"=w81:errorcluster)  [unwired: 12 in]
      n452 = call <vilib>:"DAQmx Clear Task.vi"("task in"=w84, "error in"=w83) -> ("error out"=w76:errorcluster)  [unwired: 13 in]
      n453 = call <vilib>:"DAQmx Clear Task.vi"("task in"=w82, "error in"=w81) -> ("error out"=w75:errorcluster)  [unwired: 13 in]
      n454 = Merge Errors(w76, w75, w47) -> (w73:errorcluster)
      n455 = call <vilib>:"DAQmx Clear Task.vi"("task in"=w102, "error in"=w98) -> ("error out"=w101:errorcluster)  [unwired: 13 in]
      n456 = call <vilib>:"Simple Error Handler.vi"("type of dialog (OK msg:1)"=w113, "error in (no error)"=w101) -> ("error out"=w100:errorcluster)  [unwired: 3 in, 4 out]
      n457 = Merge Errors(w100, w73, w65, w74) -> (w96:errorcluster)
      n458 = while {
        tunnel: [w267] -> w95
        tunnel: w96 -> [w267]
        stop <- w268 stop-if-true
        # "Loop to ask if the batteries are off"
        n459 = Two Button Dialog(message="Have you turned off the High voltage?", 1:"No, thank you for reminding me! I'll go do that right now!" ("button name (\"OK\")"), 2:"Yes, of course I have." ("T button name (\"OK\")")) -> (T button?=w268:bool)
      }
    }
    frame Error {
    }
  }
  "error out" <- w40
